vi "test-simple-motor-feedforward.vi"(8 "error in (no error)":errorcluster) -> (0 "error out":errorcluster, 3 "All Tests Passed":bool)   [LabVIEW 2019]
uses:
  <vilib>/Rock Robotics/WPI/ThirdParty/JAS_Junk/TrajLib/MatBuilder_Create.vi
  <vilib>/Rock Robotics/WPI/ThirdParty/JAS_Junk/TrajLib/LinearSystemId_IdentifyVelocitySystem.vi
  <vilib>/Rock Robotics/WPI/ThirdParty/JAS_Junk/TrajLib/LinearPlntInvFF_GetUff_Single.vi
  <vilib>/Rock Robotics/WPI/ThirdParty/JAS_Junk/TrajLib/MatrixHelper_Zero.vi
  <vilib>/Rock Robotics/WPI/ThirdParty/JAS_Junk/TrajLib/LinearSystem_New.vi
  <vilib>/Rock Robotics/WPI/ThirdParty/JAS_Junk/TrajLib/LinearPlntInvFF_New_Plant.vi
  <vilib>/Rock Robotics/WPI/ThirdParty/JAS_Junk/TrajLib/Trajectory_Library.lvlib
panel:
  out "Test1":dbl
  out "ErrTest0":bool
  out "Test 0":dbl
  out "Test 0\nGood":bool
  out "ErrTest1-1":bool
  out "ErrTest1-0":bool
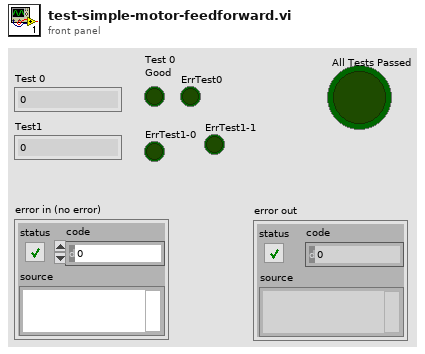
[diagram p1: front panel]
types:
  T1 = typedef "NI_Matrix.lvlib/RealMatrix.ctl" = dbl[][]
  T2 = typedef "Trajectory_Library.lvlib/LINEAR_PLANT_INV_FF.ctl" = cluster{"m_R":T1, "m_Uff":T1, "m_B":T1, "m_A":T1, "States":i32, "Inputs":i32}
  T3 = typedef "Trajectory_Library.lvlib/SIMPLE_MOTOR_FF.ctl" = cluster{"Ks":dbl, "Kv":dbl, "Ka":dbl}
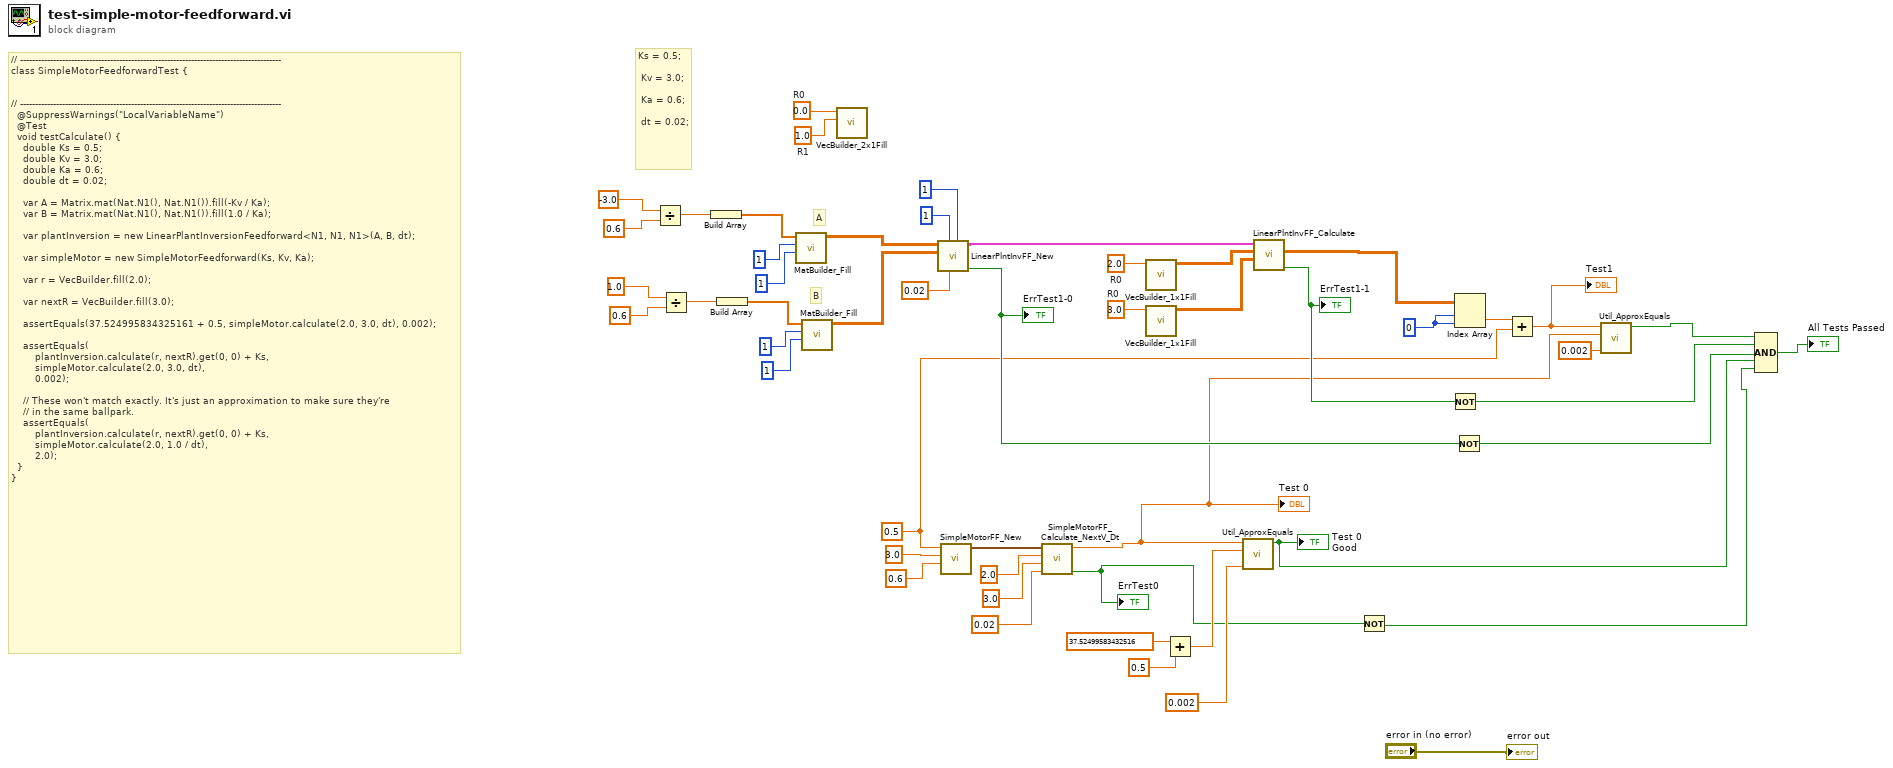
[diagram p0: block diagram]
diagram:
  w21 = 3.0  # R0
  w22 = 2.0  # R0
  w9 = 0.5 ("Ks")
  w40 = 0 ("index (row)")
  w48 = 1.0  # R1
  w47 = 0.0  # R0
  # "B"
  # "A"
  # "Ks = 0.5;\n \n Kv = 3.0;\n\n Ka = 0.6;\n\n dt = 0.02;"
  # "// ---------------------------------------------------------------------------------------\nclass SimpleMotorFeedforwardTest {\n\n\n// ---------------------------------------------------------------------------------------\n  @SuppressWarnings(\"LocalVariableName\")\n  @Test\n  void testCalculate() {\n    double Ks = 0.5;\n    double Kv = 3.0;\n    double Ka = 0.6;\n    double dt = 0.02;\n\n    var A = Matrix.mat(Nat.N1(), Nat.N1()).fill(-Kv / Ka);\n    var B = Matrix.mat(Nat.N1(), Nat.N1()).fill(1.0 / Ka);\n\n    var plantInversion = new LinearPlantInversionFeedforward<N1, N1, N1>(A, B, dt);\n\n    var simpleMotor = new SimpleMotorFeedforward(Ks, Kv, Ka);\n\n    var r = VecBuilder.fill(2.0);\n\n    var nextR = VecBuilder.fill(3.0);\n\n    assertEquals(37.524995834325161 + 0.5, simpleMotor.calculate(2.0, 3.0, dt), 0.002);\n\n    assertEquals(\n        plantInversion.calculate(r, nextR).get(0, 0) + Ks,\n        simpleMotor.calculate(2.0, 3.0, dt),\n        0.002);\n\n    // These won't match exactly. It's just an approximation to make sure they're\n    // in the same ballpark.\n    assertEquals(\n        plantInversion.calculate(r, nextR).get(0, 0) + Ks,\n        simpleMotor.calculate(2.0, 1.0 / dt),\n        2.0);\n  }\n}"
  n1 = Divide(x=-3.0, y=0.6) -> (x/y=w34:dbl)
  n2 = Divide(x=1.0, y=0.6) -> (x/y=w28:dbl)
  n3 = Build Array(w34) -> (w49:dbl[])
  n4 = Build Array(w28) -> (w29:dbl[])
  n5 = call <vilib>:"MatBuilder_Fill.vi"("Columns"=1, "Rows"=1, "Value List"=w49) -> ("output matrix"=w44:T1)  [unwired: 8 in]
  n6 = call <vilib>:"MatBuilder_Fill.vi"("Columns"=1, "Rows"=1, "Value List"=w29) -> ("output matrix"=w25:T1)  [unwired: 8 in]
  n7 = call <vilib>:"VecBuilder_2x1Fill.vi"("R1"=w48, "R0"=w47) -> ()  [unwired: 9 in, 1 out]
  n8 = call <vilib>:"LinearPlntInvFF_New.vi"("States"=1, "dT_Seconds"=0.02, "Inputs"=1, "B"=w25, "A"=w44) -> ("Error"=w37:bool, "Linear Plnt Inversion FF"=w42:T2)  [unwired: 5 in]
  "ErrTest1-0" <- w37
  n9 = call <vilib>:"SimpleMotorFF_New.vi"("Ka"=0.6, "Kv"=3.0, "Ks"=w9) -> ("SIMPLE_MOTOR_FF"=w18:T3)  [unwired: 8 in]
  n10 = call <vilib>:"SimpleMotorFF_Calculate_NextV_Dt.vi"("dT_Sec"=0.02, "NextVel_SP"=3.0 ("Accel"), "Vel_SP"=2.0 ("Vel"), "SIMPLE_MOTOR_FF"=w18) -> ("Error"=w4:bool, "FeedForward"=w7:dbl)  [unwired: 6 in]
  "Test 0" <- w7
  "ErrTest0" <- w4
  n11 = call <vilib>:"VecBuilder_1x1Fill.vi"("R0_C0"=w22) -> ("output matrix"=w20:T1)  [unwired: 10 in]
  n12 = call <vilib>:"VecBuilder_1x1Fill.vi"("R0_C0"=w21) -> ("output matrix"=w19:T1)  [unwired: 10 in]
  n13 = Add(x=37.52499583432516, y=0.5) -> (x+y=w13:dbl)
  n14 = call <vilib>:"Util_ApproxEquals.vi"("Tolerance"=0.002, "Value 2"=w13, "Value 1"=w7) -> ("ApproxEquals"=w3:bool)  [unwired: 8 in]
  "Test 0\nGood" <- w3
  n15 = call <vilib>:"LinearPlntInvFF_Calculate.vi"("NextR"=w19, "R"=w20, "Input Linear Plant Inv FF"=w42) -> ("Error"=w38:bool, "Uff"=w41:T1)  [unwired: 6 in, 1 out]
  "ErrTest1-1" <- w38
  n16 = Not(x=w4) -> (.not. x?=w2:bool)
  n17 = Not(x=w38) -> (.not. x?=w39:bool)
  n18 = Not(x=w37) -> (.not. x?=w36:bool)
  n19 = Index Array(array=w41, index (row)=w40, index (col)=w40) -> (element=w10:dbl)
  n20 = Add(x=w10, y=w9) -> (x+y=w8:dbl)
  "Test1" <- w8
  n21 = call <vilib>:"Util_ApproxEquals.vi"("Tolerance"=0.002, "Value 2"=w7, "Value 1"=w8) -> ("ApproxEquals"=w5:bool)  [unwired: 8 in]
  n22 = Compound Arithmetic op=AND(w5, w39, w36, w3, w2) -> (→"All Tests Passed":bool)
  "error out" <- "error in (no error)"
